vi "Brain.vi"() -> ()   [LabVIEW 2017]
uses:
  <vilib>/OPCUA/controls/NodeId.ctl
  <vilib>/OPCUA/controls/Write Status.ctl
  <vilib>/Utility/file.llb/Read Delimited Spreadsheet (string).vi
  <vilib>/Utility/file.llb/Write Delimited Spreadsheet (string).vi
  <vilib>/OPCUA/client/Multiple Write Double Array.vi
  <vilib>/OPCUA/client/Multiple Write Bool Array.vi
  <vilib>/Utility/file.llb/Write Delimited Spreadsheet (DBL).vi
  <resource>/objmgr/ni.dex.rc
  <vilib>/OPCUA/NI OPC UA Client.lvlib
panel:
  in  "VFD Stop":bool
  in  "Shutdown":bool
  out "Remote VI Error Messages":string
  in  "Node Status":u32
  in  "Time Stamp":timestamp
  in  "Error In":errorcluster
  out "Error Out":errorcluster
  in  "Stop DAQ":bool
  out "DAQ?":bool
  out "Available Elements for Reading":i32
  out "Number of Disconnections":u32
  out "System Loop Time (ms)":u32
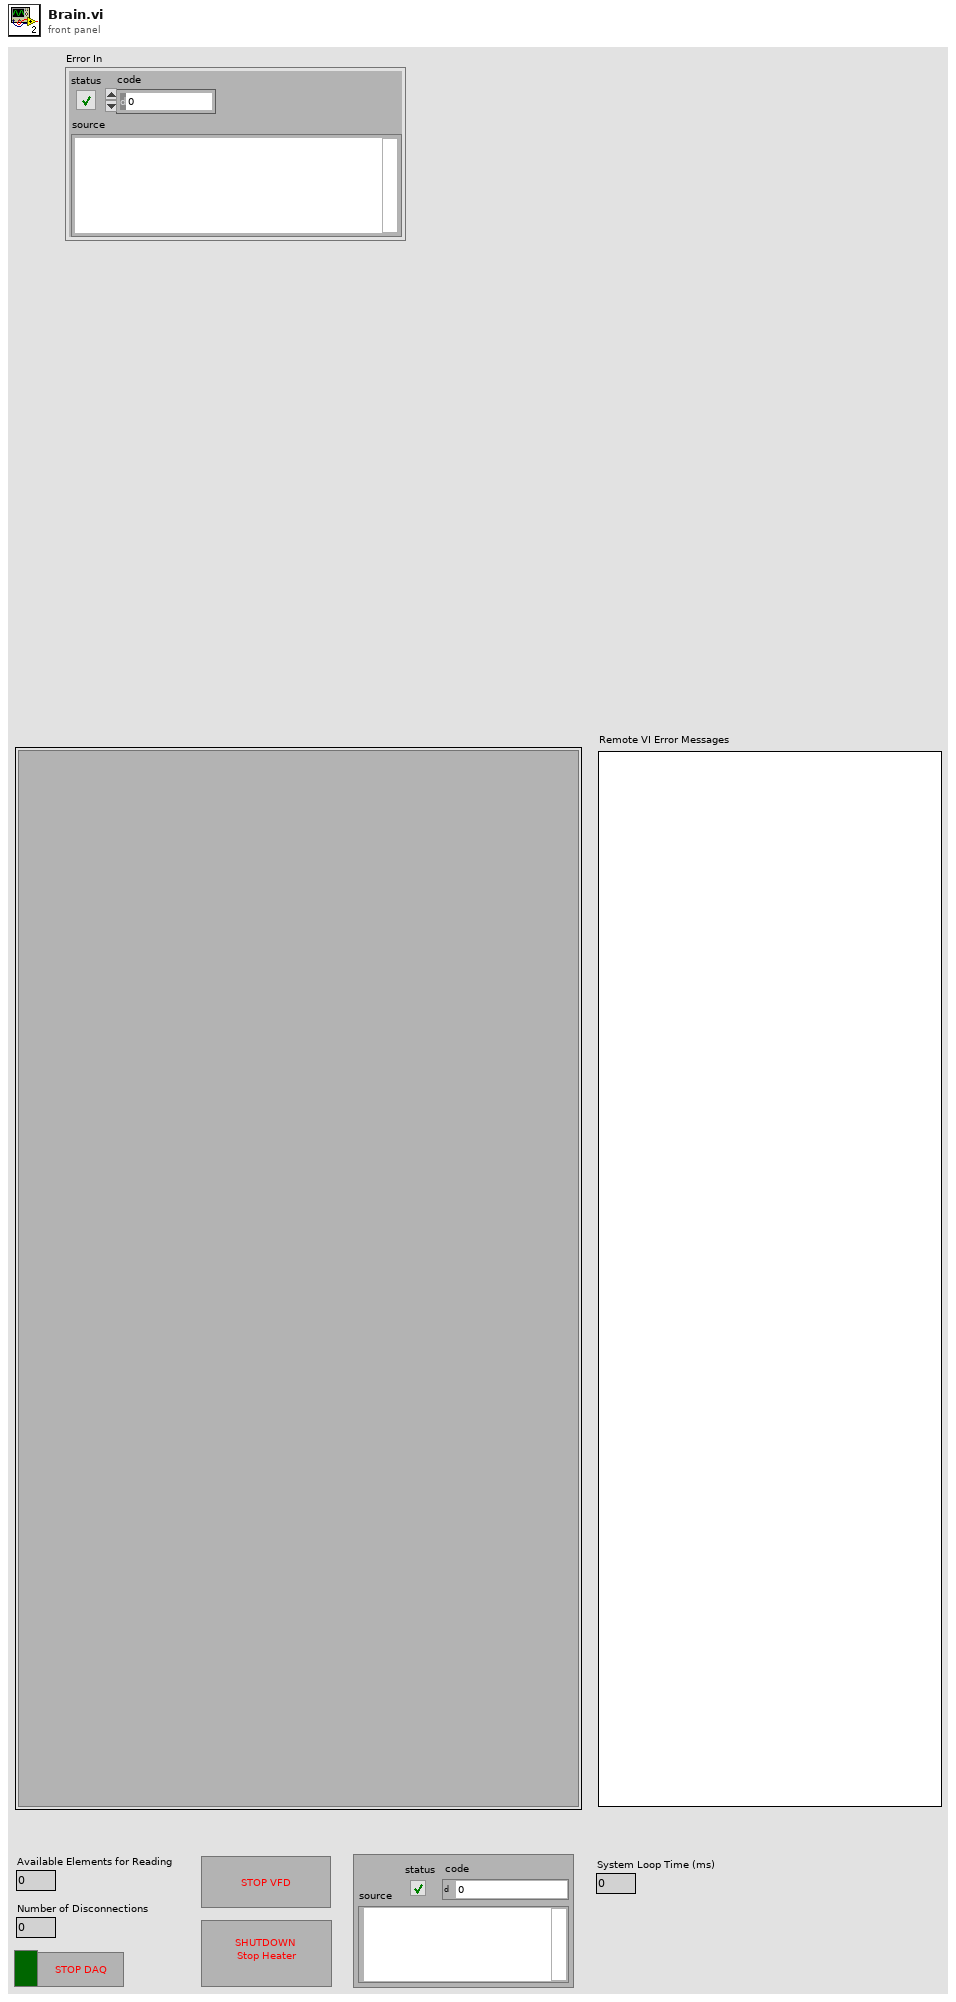
[diagram p1: front panel]
types:
  T1 = typedef "OPC UA Client Refnum.ctl" = refnum<k21>
  T2 = typedef "NodeId.ctl" = string
  T3 = typedef "Write Status.ctl" = u32
  T4 = cluster{"node ID":T2, "value":bool[], "timestamp (current time)":timestamp, "node status":T3}
  T5 = cluster{"node ID":T2, "value":dbl[], "timestamp (current time)":timestamp, "node status":T3}
  T6 = cluster{"node ID":T2, "value":dbl[], "timestamp (current time)":timestamp, "node status":T3}[]
  T7 = cluster{"node ID":T2, "value":bool[], "timestamp (current time)":timestamp, "node status":T3}[]
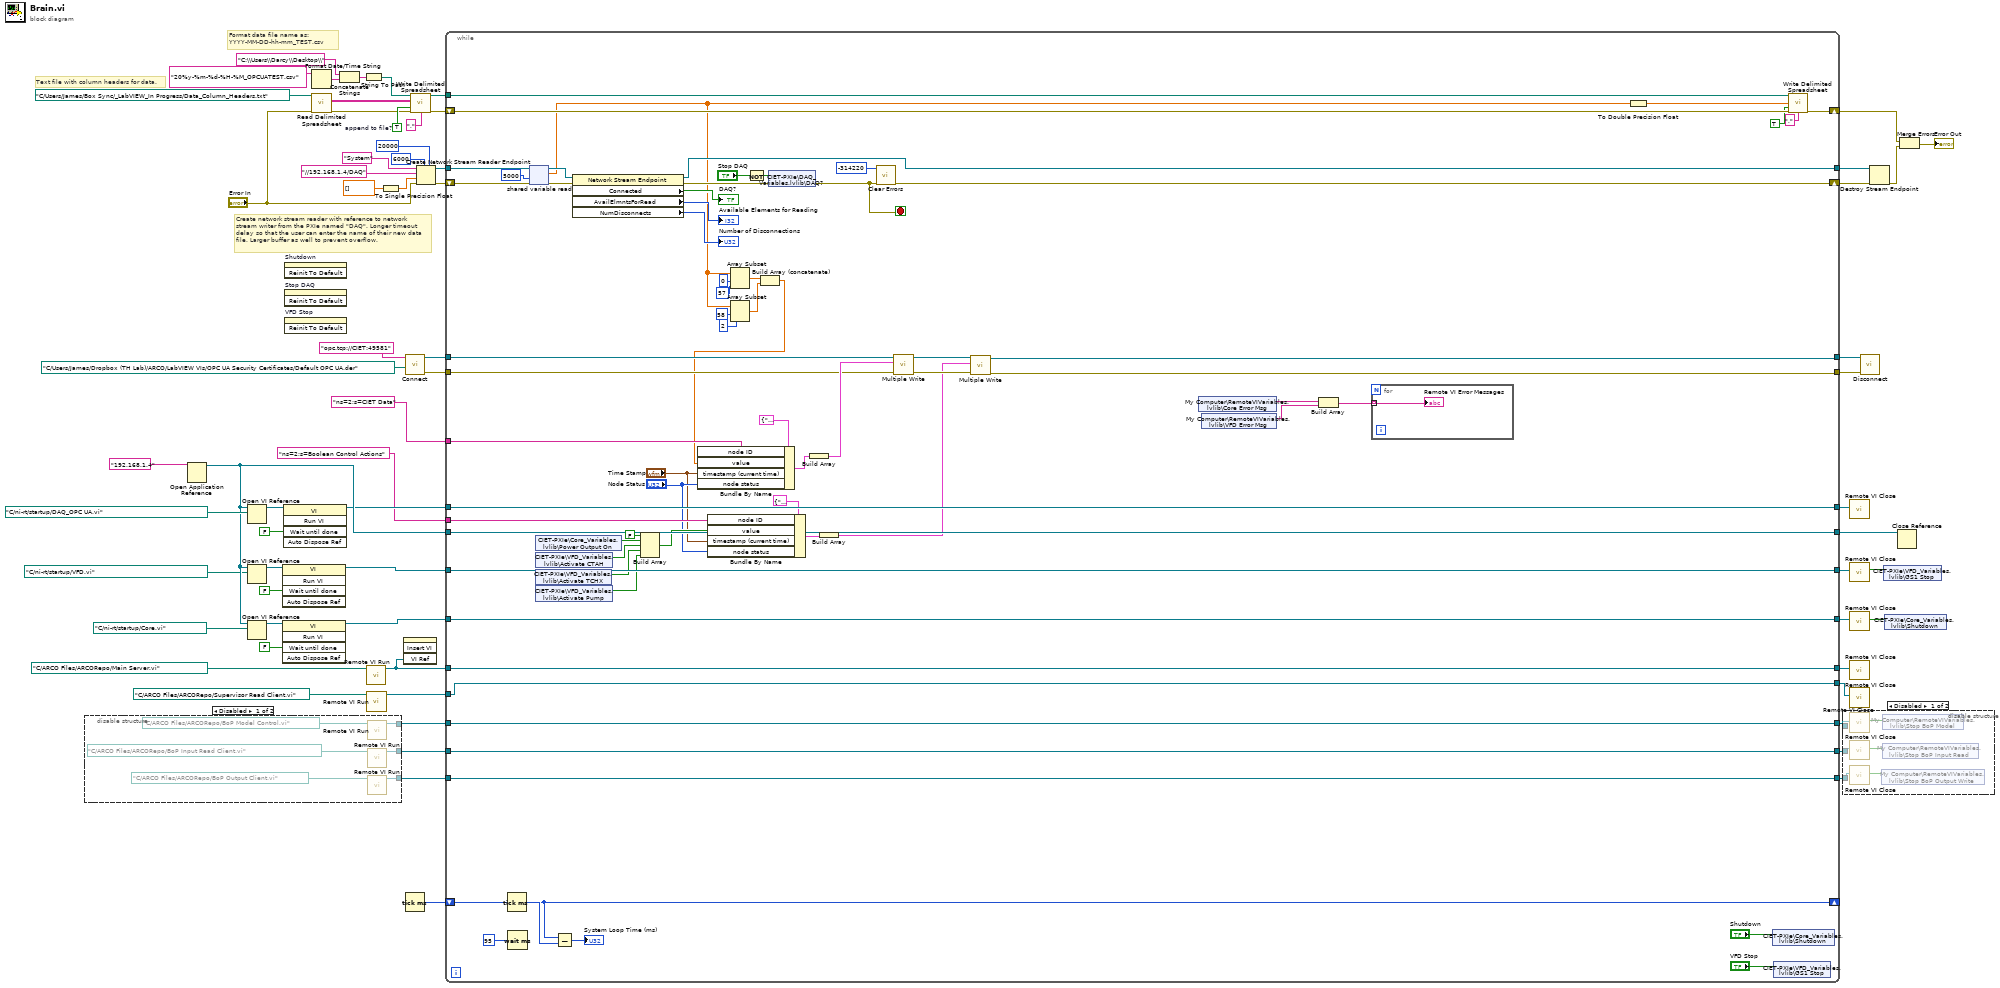
[diagram p0: block diagram]
diagram:
  w54 = TRUE  # append to file?
  # "Format data file name as:\nYYYY-MM-DD-hh-mm_TEST.csv"
  # "Create network stream reader with reference to network\nstream writer from the PXIe named \"DAQ\". Longer timeout\ndelay so that the user can enter the name of their new data\nfile. Larger buffer as well to prevent overflow."
  # "Text file with column headers for data."
  n1 = disable-structure shown="Disabled" {
    disable-tunnel: [w70 _] -> w6
    disable-tunnel: [w69 _] -> w4
    disable-tunnel: [w68 _] -> w2
    frame Disabled {
      n2 = call "Remote VI Run.vi"("VI Path"=path "C:/ARCO Files/ARCORepo/BoP Model Control.vi" ("vi path")) -> ("VI Reference"=w70:refnum<vi>)  [unwired: 10 in]
      n3 = call "Remote VI Run.vi"("VI Path"=path "C:/ARCO Files/ARCORepo/BoP Input Read Client.vi" ("vi path")) -> ("VI Reference"=w69:refnum<vi>)  [unwired: 10 in]
      n4 = call "Remote VI Run.vi"("VI Path"=path "C:/ARCO Files/ARCORepo/BoP Output Client.vi" ("vi path")) -> ("VI Reference"=w68:refnum<vi>)  [unwired: 10 in]
    }
    frame Enabled {
    }
  }
  n5 = Open Application Reference(11:"192.168.1.4" ("machine name (\"\":  open local reference)")) -> (3:w25:refnum<vi>)  [unwired: 3 in, 1 out]
  n6 = Open VI Reference(application reference (local)=w25, vi path=path "C:/ni-rt/startup/DAQ_OPC UA.vi") -> (vi reference=w22:refnum<vi>)  [unwired: 4 in, 1 out]
  n7 = Open VI Reference(application reference (local)=w25, vi path=path "C:/ni-rt/startup/VFD.vi") -> (vi reference=w20:refnum<vi>)  [unwired: 4 in, 1 out]
  n8 = Open VI Reference(application reference (local)=w25, vi path=path "C:/ni-rt/startup/Core.vi") -> (vi reference=w18:refnum<vi>)  [unwired: 4 in, 1 out]
  n9 = invoke class="VI" method="Run VI"(reference=w20, "Wait until done"=FALSE ("Wait Until Done")) -> (reference out=w19:refnum<vi>)  [unwired: 3 in, 4 out]
  n10 = invoke class="VI" method="Run VI"(reference=w18, "Wait until done"=FALSE ("Wait Until Done")) -> (reference out=w17:refnum<vi>)  [unwired: 3 in, 4 out]
  n11 = invoke class="VI" method="Run VI"(reference=w22, "Wait until done"=FALSE ("Wait Until Done")) -> (reference out=w21:refnum<vi>)  [unwired: 3 in, 4 out]
  n12 = invoke on="Shutdown" class="Bool (strict)" method="Reinit To Default"() -> ()  [unwired: 3 in, 3 out]
  n13 = invoke on="Stop DAQ" class="Bool (strict)" method="Reinit To Default"() -> ()  [unwired: 3 in, 3 out]
  n14 = invoke on="VFD Stop" class="Bool (strict)" method="Reinit To Default"() -> ()  [unwired: 3 in, 3 out]
  n15 = Format Date/Time String(time format string (%c)="20%y-%m-%d-%H-%M_OPCUATEST.csv") -> (date/time string=w44:string)  [unwired: 2 in]
  n16 = call-poly <vilib>:"Read Delimited Spreadsheet.vi"("file path (dialog if empty)"=path "C:/Users/James/Box Sync/_LabVIEW_In Progress/Data_Column_Headers.txt", "error in (no error)"="Error In") -> ("all rows"=w57:string[][], "error out"=w52:errorcluster)  [unwired: 8 in, 4 out]
  n17 = Concatenate Strings("C:\\Users\\Darcy\\Desktop\\" ("string"), w44) -> (w46:string)
  n18 = String To Path(string=w46) -> (path=w43:path)
  n19 = call "Remote VI Run.vi"("VI Path"=path "C:/ARCO Files/ARCORepo/Main Server.vi" ("vi path")) -> ("VI Reference"=w27:refnum<vi>)  [unwired: 10 in]
  n20 = call "Remote VI Run.vi"("VI Path"=path "C:/ARCO Files/ARCORepo/Supervisor Read Client.vi" ("vi path")) -> ("VI Reference"=w8:refnum<vi>)  [unwired: 10 in]
  n21 = To Single Precision Float(number=dbl[] []) -> (single precision float=w65:sgl[])
  n22 = invoke on="Sub Panel" class="SubPnl" method="Insert VI"("VI Ref"=w27) -> ()  [unwired: 3 in, 4 out]
  n23 = call <vilib>:"Connect.vi"("client certificate file"=path "C:/Users/James/Dropbox (TH Lab)/ARCO/LabVIEW VIs/OPC UA Security Certificates/Default OPC UA.der", "server endpoint URL"="opc.tcp://CIET:49581") -> ("error out"=w37:errorcluster, "OPC UA client refnum out"=w38:T1)  [unwired: 7 in, 1 out]
  n24 = Tick Count (ms)() -> (millisecond timer value=w41:u32)
  n25 = call-poly <vilib>:"Write Delimited Spreadsheet.vi"("file path (dialog if empty)"=w43, "2D data"=w57, "append to file? (new file:F)"=w54, "error in (no error)"=w52, "delimiter (\\t)"=",") -> ("new file path (Not A Path if cancelled)"=w53:path, "error out"=w51:errorcluster)  [unwired: 9 in]
  n26 = Create Network Stream Reader Endpoint(5:20000 ("timeout in ms (-1)"), 7:6000 ("reader buffer size"), 8:"Error In", 9:w65, 10:"//192.168.1.4/DAQ" ("writer url"), 11:"System" ("reader name")) -> (0:w62:errorcluster, 3:w61:refnum<k21>)  [unwired: 1 in]
  n27 = while {
    shift-right: [w131] -> w60
    shift-left: w62 -> [w139]
    tunnel: w61 -> [w140]
    tunnel: [w130] -> w59
    tunnel: w53 -> [w126]
    shift-right: [w124] -> w50
    shift-left: w51 -> [w125]
    shift-right: [w119] -> _
    shift-left: w41 -> [w120]
    tunnel: w38 -> [w114]
    tunnel: w37 -> [w113]
    tunnel: "ns=2;s=CIET Data" -> [w112]
    tunnel: [w79] -> w35
    tunnel: [w78] -> w34
    tunnel: w21 -> [w111]
    tunnel: [w111] -> w32
    tunnel: w25 -> [w110]
    tunnel: [w110] -> w31
    tunnel: w19 -> [w109]
    tunnel: [w109] -> w30
    tunnel: w17 -> [w108]
    tunnel: [w108] -> w29
    tunnel: w27 -> [w107]
    tunnel: [w107] -> w28
    tunnel: "ns=2;s=Boolean Control Actions" -> [w94]
    tunnel: w8 -> [w77]
    tunnel: [w77] -> w7
    tunnel: w6 -> [w76]
    tunnel: [w76] -> w5
    tunnel: w4 -> [w75]
    tunnel: [w75] -> w3
    tunnel: w2 -> [w74]
    tunnel: [w74] -> w1
    stop <- w129 stop-if-true
    n28 = Tick Count (ms)() -> (millisecond timer value=w119:u32)
    n29 = Wait (ms)(milliseconds to wait=u32 95) -> ()  [unwired: 1 out]
    n30 = shared-variable-read(w140, w139, 5000 ("timeout ms (-1)")) -> (w136:refnum<k21>, w134:errorcluster, w83:sgl[])  [unwired: 1 out]
    n31 = shared-variable "CIET-PXIe\\Core_Variables.lvlib\\Power Output On"() -> (w100:bool)  [unwired: 1 in, 1 out]
    n32 = shared-variable "CIET-PXIe\\VFD_Variables.lvlib\\Activate CTAH"() -> (w99:bool)  [unwired: 1 in, 1 out]
    n33 = shared-variable "CIET-PXIe\\VFD_Variables.lvlib\\Activate TCHX"() -> (w98:bool)  [unwired: 1 in, 1 out]
    n34 = shared-variable "CIET-PXIe\\VFD_Variables.lvlib\\Activate Pump"() -> (w97:bool)  [unwired: 1 in, 1 out]
    n35 = Subtract(x=w119, y=w120) -> (x-y=→"System Loop Time (ms)":u32)
    n36 = property class="Network Stream Endpoint"(reference=w136, error in=w134) -> (reference out=w130:refnum<k21>, error out=w135:errorcluster, "Connected"=→"DAQ?":bool, "AvailElmntsForRead"=→"Available Elements for Reading":i32, "NumDisconnects"=→"Number of Disconnections":u32)
    n37 = Build Array(FALSE ("element"), w100, w99, w98, w97) -> (w96:bool[])
    n38 = Bundle By Name(cluster=T4 {"node ID"="", "value"=[], "timestamp (current time)"=timestamp(0 s since 1904-01-01), "node status"=0} ("request"), "node ID"=w94, "value"=w96, "timestamp (current time)"="Time Stamp", "node status"="Node Status") -> (w101:T4)
    n39 = Array Subset(array=w83, index=0, length=57) -> (w86:sgl[])
    n40 = Array Subset(array=w83, index=58, length=2) -> (w82:sgl[])
    n41 = Not(x="Stop DAQ") -> (.not. x?=w138:bool)
    n42 = Build Array (concatenate)(w86, w82) -> (w80:sgl[])
    n43 = Bundle By Name(cluster=T5 {"node ID"="", "value"=[], "timestamp (current time)"=timestamp(0 s since 1904-01-01), "node status"=0} ("request"), "node ID"=w112, "value"=w80, "timestamp (current time)"="Time Stamp", "node status"="Node Status") -> (w116:T5)
    n44 = shared-variable "CIET-PXIe\\DAQ_Variables.lvlib\\DAQ?"(w138, error in=w135) -> (error out=w129:errorcluster)
    n45 = Build Array(w116) -> (w115:T6)
    n46 = Build Array(w101) -> (w89:T7)
    n47 = call <vilib>:"Clear Errors.vi"("error in (no error)"=w129, "specific error code to clear (0: all)"=-314220) -> ("error out"=w131:errorcluster)  [unwired: 4 in, 1 out]
    n48 = call-poly <vilib>:"Multiple Write.vi"("error in (no error)"=w113, "requests"=w115, "OPC UA client refnum in"=w114) -> ("error out"=w91:errorcluster, "OPC UA client refnum out"=w92:T1)  [unwired: 5 in, 2 out]
    n49 = call-poly <vilib>:"Multiple Write.vi"("error in (no error)"=w91, "requests"=w89, "OPC UA client refnum in"=w92) -> ("error out"=w78:errorcluster, "OPC UA client refnum out"=w79:T1)  [unwired: 5 in, 2 out]
    n50 = shared-variable "My Computer\\RemoteVIVariables.lvlib\\Core Error Msg"() -> (w106:string)  [unwired: 1 in, 1 out]
    n51 = shared-variable "My Computer\\RemoteVIVariables.lvlib\\VFD Error Msg"() -> (w105:string)  [unwired: 1 in, 1 out]
    n52 = Build Array(w106, w105) -> (w104:string[])
    n53 = for {
      tunnel: w104 -> [w143] mode=indexing
      "Remote VI Error Messages" <- w143
    }
    n54 = To Double Precision Float(number=w83) -> (double precision float=w121:dbl[])
    n55 = shared-variable "CIET-PXIe\\Core_Variables.lvlib\\Shutdown"("Shutdown") -> ()  [unwired: 1 in, 1 out]
    n56 = shared-variable "CIET-PXIe\\VFD_Variables.lvlib\\GS1 Stop"("VFD Stop") -> ()  [unwired: 1 in, 1 out]
    n57 = call-poly <vilib>:"Write Delimited Spreadsheet.vi"("file path (dialog if empty)"=w126, "1D data"=w121, "append to file? (new file:F)"=TRUE, "error in (no error)"=w125, "delimiter (\\t)"="," ("delimiter (\\t)")) -> ("error out"=w124:errorcluster)  [unwired: 9 in, 1 out]
  }
  n58 = disable-structure shown="Disabled" {
    disable-tunnel: w5 -> [w149 _]
    disable-tunnel: w3 -> [w148 _]
    disable-tunnel: w1 -> [w147 _]
    frame Disabled {
      n59 = call "Remote VI Close.vi"("reference"=w149) -> ("SubVI Stop"=w145:bool)  [unwired: 10 in]
      n60 = call "Remote VI Close.vi"("reference"=w148) -> ("SubVI Stop"=w144:bool)  [unwired: 10 in]
      n61 = call "Remote VI Close.vi"("reference"=w147) -> ("SubVI Stop"=w146:bool)  [unwired: 10 in]
      n62 = shared-variable "My Computer\\RemoteVIVariables.lvlib\\Stop BoP Output Write"(w146) -> ()  [unwired: 1 in, 1 out]
      n63 = shared-variable "My Computer\\RemoteVIVariables.lvlib\\Stop BoP Model"(w145) -> ()  [unwired: 1 in, 1 out]
      n64 = shared-variable "My Computer\\RemoteVIVariables.lvlib\\Stop BoP Input Read"(w144) -> ()  [unwired: 1 in, 1 out]
    }
    frame Enabled {
    }
  }
  n65 = call "Remote VI Close.vi"("reference"=w32) -> ()  [unwired: 10 in, 1 out]
  n66 = call "Remote VI Close.vi"("reference"=w30) -> ("SubVI Stop"=w12:bool)  [unwired: 10 in]
  n67 = call "Remote VI Close.vi"("reference"=w29) -> ("SubVI Stop"=w13:bool)  [unwired: 10 in]
  n68 = call "Remote VI Close.vi"("reference"=w28) -> ()  [unwired: 10 in, 1 out]
  n69 = call "Remote VI Close.vi"("reference"=w7) -> ()  [unwired: 10 in, 1 out]
  n70 = call <vilib>:"Disconnect.vi"("error in (no error)"=w34, "OPC UA client refnum in"=w35) -> ()  [unwired: 9 in, 1 out]
  n71 = Destroy Stream Endpoint(8:w60, 11:w59) -> (0:w49:errorcluster)
  n72 = shared-variable "CIET-PXIe\\VFD_Variables.lvlib\\GS1 Stop"(w12) -> ()  [unwired: 1 in, 1 out]
  n73 = shared-variable "CIET-PXIe\\Core_Variables.lvlib\\Shutdown"(w13) -> ()  [unwired: 1 in, 1 out]
  n74 = Close Reference(reference=w31) -> ()  [unwired: 1 in, 1 out]
  n75 = Merge Errors(w50, w49) -> (→"Error Out":errorcluster)
